vi "CD Address Lookup Table Initialize.vi"(8 "error in (no error)":errorcluster) -> (0 "error out":errorcluster {"code" min=0 max=0}, 3 "ref":T1)   [LabVIEW 2013, in "J1939.lvlib"]
uses:
  LUTs/J1939 Address Table Reference.ctl
  LUTs/J1939 Address Lookup Table Action.ctl
  J1939.lvlib
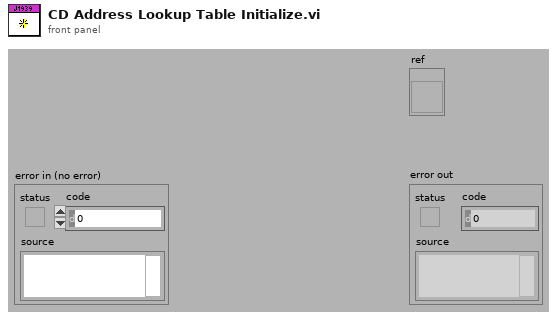
[diagram p1: front panel]
types:
  T1 = typedef "J1939.lvlib/J1939 Address Table Reference.ctl" = refnum<vi>
  T2 = typedef "J1939.lvlib/J1939 Address Lookup Table Action.ctl" = enum16{"Initialize", "Add", "Get", "Remove", "Get All"}
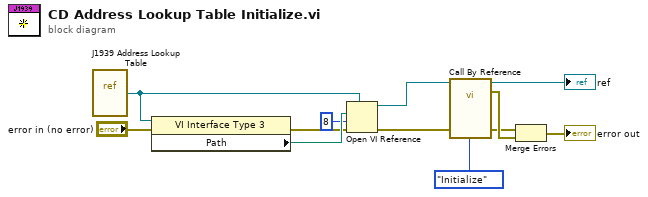
[diagram p0: block diagram]
diagram:
  n1 = vi-ref "J1939 Address Lookup Table.vi"() -> (w12:refnum<vi>)
  n2 = property class="VI Interface Type 3"(reference=w12, error in="error in (no error)") -> (error out=w9:errorcluster, "Path"=w11:path)  [unwired: 1 out]
  n3 = Open VI Reference(type specifier VI Refnum (for type only)=w12, vi path=w11, options=8, error in (no error)=w9) -> (vi reference=w8:refnum<vi>, error out=w4:errorcluster)  [unwired: 2 in]
  n4 = call-by-ref "?"(reference=w8, "Action"=J1939_Address_Lookup_Table_Action."Initialize", "error in (no error)"=w4) -> (reference out=→"ref":refnum<vi>, error out=w7:errorcluster, 0:"error out"=w3:errorcluster)  [unwired: 7 in, 3 out]
  n5 = Merge Errors(w3, w7) -> (→"error out":errorcluster)
